vi "GPI-Movie merge.vi"() -> ()   [LabVIEW 2011]
doc: "Makes merged pseudo-color stills or movies from microscope images collected at two different wavelengths. Can handle either simultaneous or sequential multiwavelength acquisitions. The program uses the Matlab image registration tools to do the image alignments; these tools require the user to pick control points manually by mouse clicking. The images used to pick control points can be the images of the experiment or separate control images of a registration sample. The program handles tiffs or tiff stacks for stills; movies must be tiff stacks."
panel:
  in  "About":bool
  in  "Make a Movie":bool
  in  "Read Alignment Info from File":bool
  in  "Save Alignment Info to File":bool
  in  "View Alignment Images and Select Control Points":bool
  out "error out":errorcluster
  in  "Make a Merged Still Image and adjust intensities":bool
  in  "stop":bool
  in  "error in (no error)":errorcluster
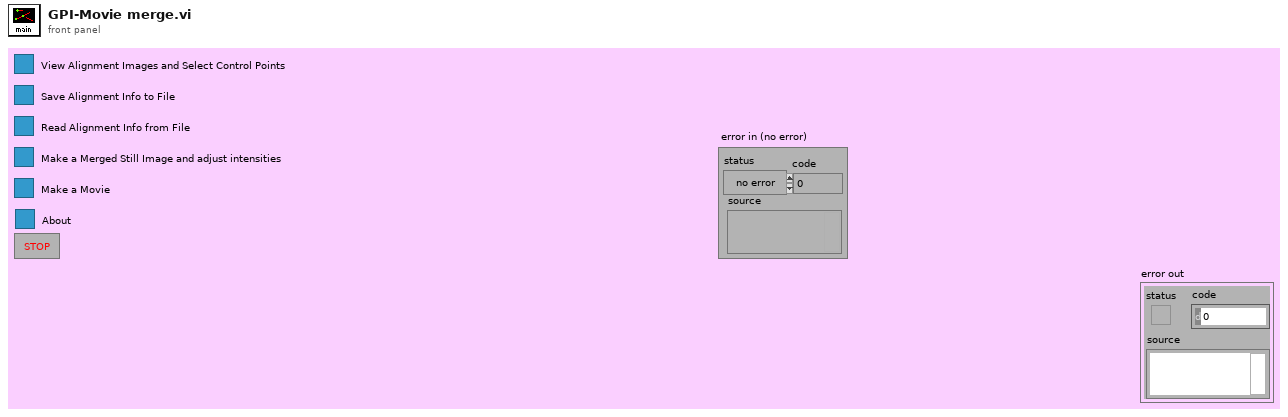
[diagram p1: front panel]
types:
  T1 = cluster{"File name":path, "TIFF stack?":bool, "Frame # if stack?":u32}[]
  T2 = typedef "IMAQ Image.ctl" = refnum<image>
  T3 = cluster{"Image Type":u32, "Image":T2, "Initialized?":bool, "Window Title":string, "Auto resize?":bool, "Auto position?":bool, "Autoscale?":bool, "Black/White Levels":cluster{ext, ext}, "Scale Min":ext, "Scale Max":ext}[]
  T4 = enum32{"existing file", "new file", "new or existing file", "existing dir", "new dir", "new or existing dir", "existing file (use LLBs)", "new file (use LLBs)", "new or existing file (use LLBs)", "new or existing file or directory (use LLBs)"}
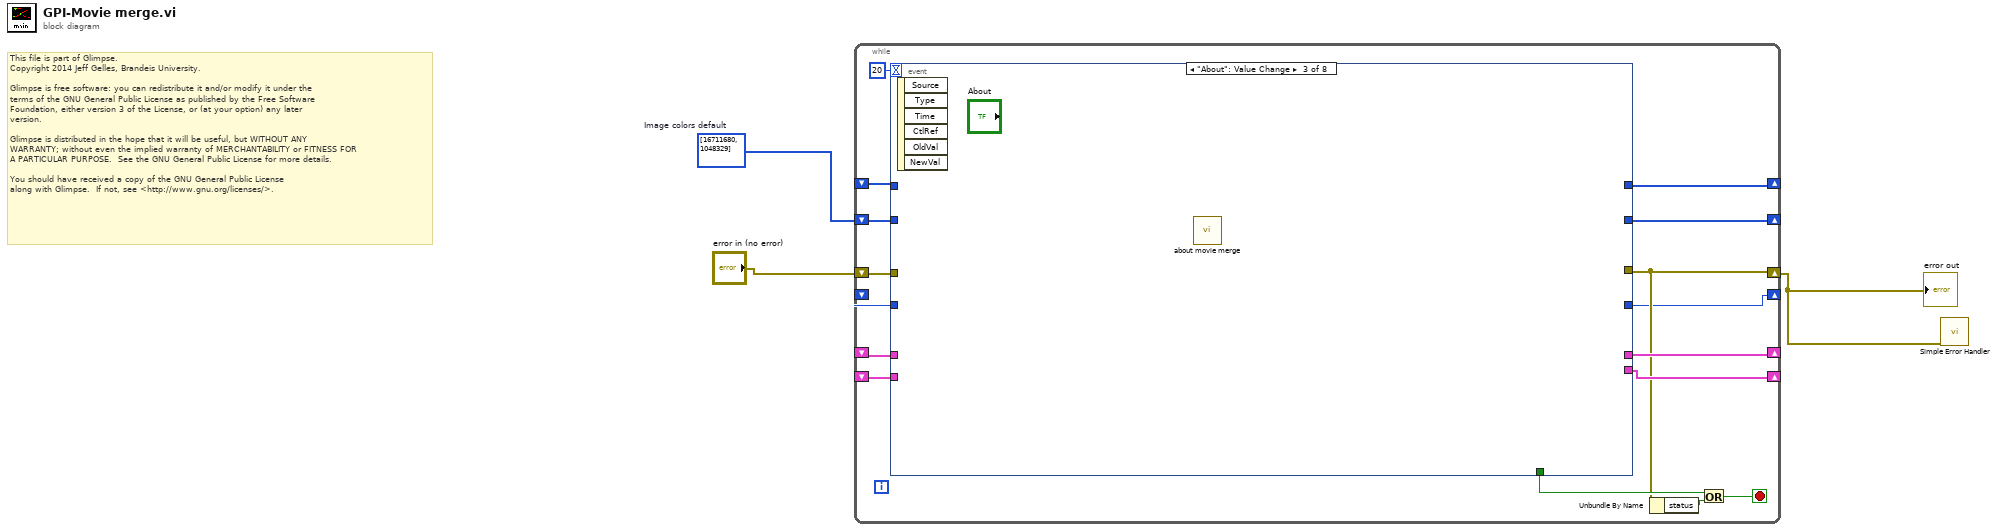
[diagram p0: block diagram]
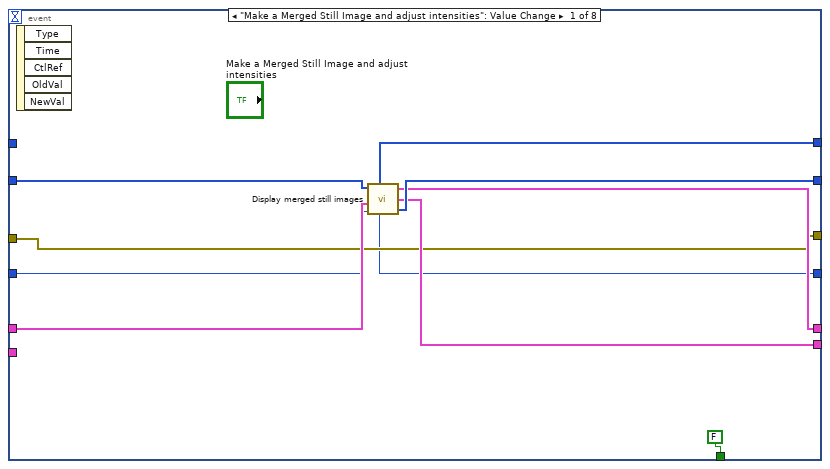
[diagram p2: hidden frame]
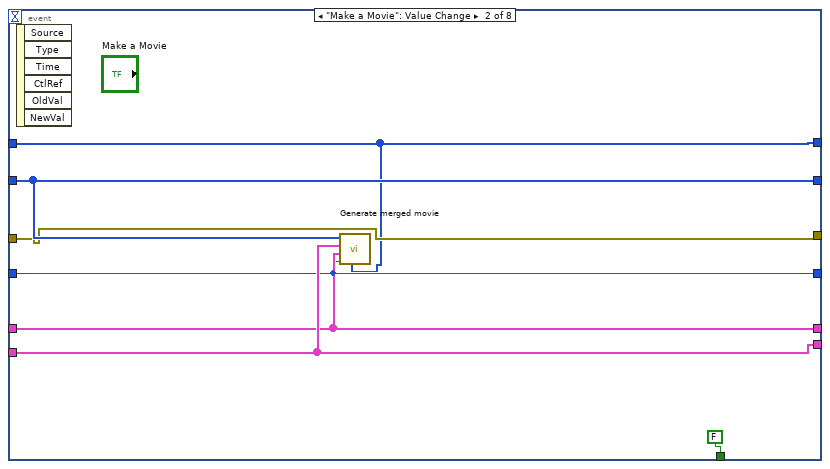
[diagram p3: hidden frame]
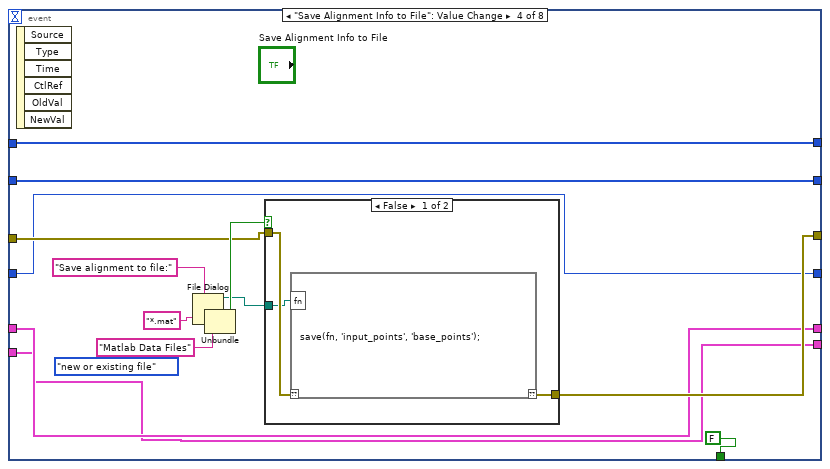
[diagram p4: hidden frame]
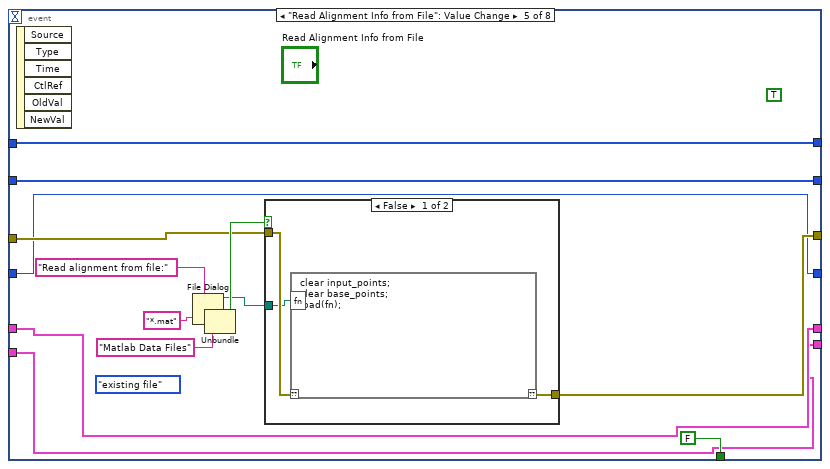
[diagram p6: hidden frame]
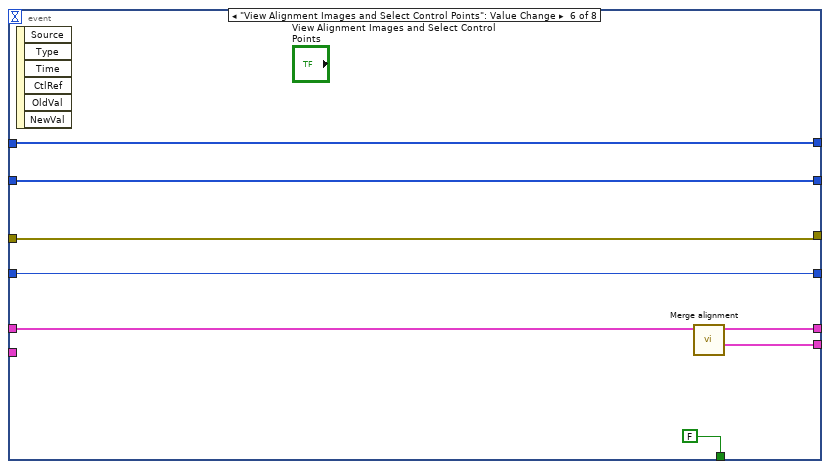
[diagram p8: hidden frame]
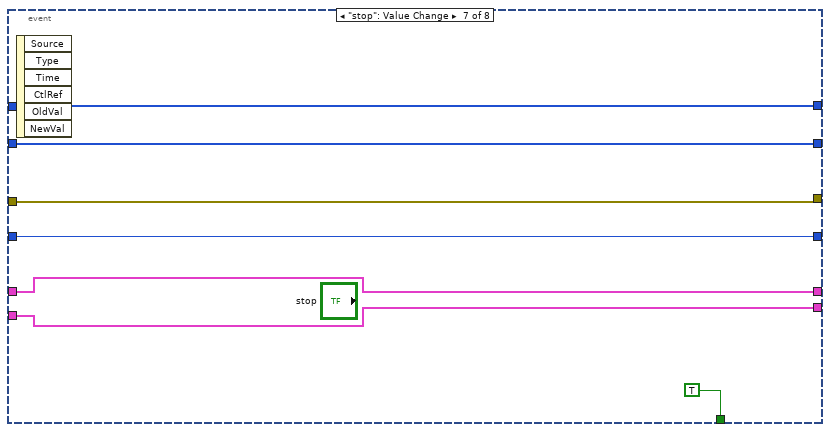
[diagram p9: hidden frame]
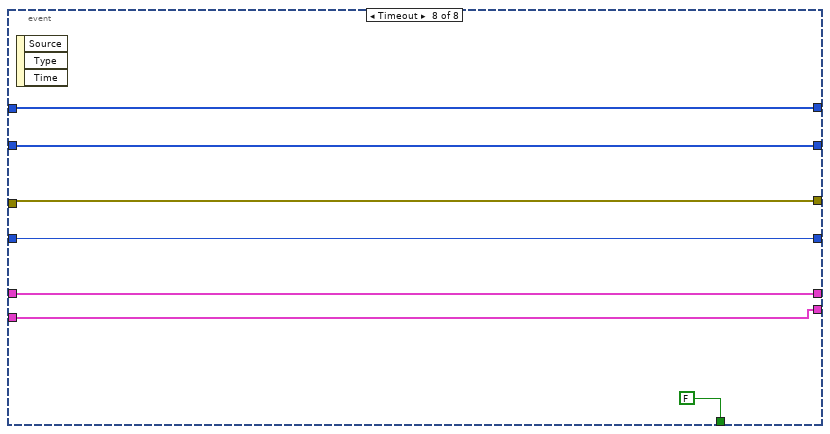
[diagram p10: hidden frame]
diagram:
  w1 = u32[] [16711680, 1048329]  # Image colors default
  # "This file is part of Glimpse. \nCopyright 2014 Jeff Gelles, Brandeis University.    \n\nGlimpse is free software: you can redistribute it and/or modify it under the \nterms of the GNU General Public License as published by the Free Software \nFoundation, either version 3 of the License, or (at your option) any later \nversion.\n\nGlimpse is distributed in the hope that it will be useful, but WITHOUT ANY \nWARRANTY; without even the implied warranty of MERCHANTABILITY or FITNESS FOR \nA PARTICULAR PURPOSE.  See the GNU General Public License for more details.\n\nYou should have received a copy of the GNU General Public License\nalong with Glimpse.  If not, see <http://www.gnu.org/licenses/>."
  n1 = while {
    shift-right: [w8] -> w2
    shift-left: "error in (no error)" -> [w15]
    shift-right: [w14] -> _
    shift-left: _ -> [w12]
    shift-right: [w13] -> _
    shift-left: _ -> [w11]
    shift-right: [w10] -> _
    shift-left: w1 -> [w9]
    shift-right: [w6] -> _
    shift-left: _ -> [w7]
    shift-right: [w5] -> _
    shift-left: _ -> [w4]
    stop <- w19 stop-if-true
    n2 = event shown="[2] \"About\": Value Change" {
      selector: _ -> [_ _ _ _ _ _ _ _]
      dyn-events: _ -> [_ _ _ _ _ _ _ _]
      timeout: 20 -> [_ _ _ _ _ _ _ _]
      tunnel: [FALSE ("stop") FALSE ("stop") _ FALSE ("stop") FALSE ("stop") FALSE ("stop") TRUE FALSE ("stop")] -> w18
      tunnel: w15 -> [w23 w33 _ w43 w61 w75 w86 w93]
      tunnel: [w23 w33 _ w45 w63 w75 w86 w93] -> w8
      tunnel: [w26 w35 _ w42 w60 w79 w85 w91] -> w14
      tunnel: [w25 w36 _ w41 w59 w78 w84 w90] -> w13
      tunnel: w12 -> [w24 w35 _ w42 w60 w77 w85 w91]
      tunnel: w11 -> [_ w36 _ w41 w59 _ w84 w90]
      tunnel: [w28 w34 _ w40 w58 w76 w83 w92] -> w10
      tunnel: w9 -> [w27 w34 _ w40 w58 w76 w83 w92]
      tunnel: w7 -> [w21 w32 _ w39 w57 w74 w82 w89]
      tunnel: [w22 w32 _ w39 w57 w74 w82 w89] -> w6
      tunnel: [w20 w31 _ w38 w56 w73 w81 w88] -> w5
      tunnel: w4 -> [_ w31 _ w38 w56 w73 w81 w88]
      event "Make a Merged Still Image and adjust intensities": Value Change {
        n3 = event-data() -> ()  [unwired: 6 out]
        n4 = call "Display merged still images.vi"("Image colors"=w27, "Image info"=w24, "Transform"=w21) -> ("ROI Out"=w20:i32[], "Transform out"=w22:u16, "Image info Out"=w26:T1, "Display info out"=w25:T3, "Image colors out"=w28:u32[])  [unwired: 1 out]
      }
      event "Make a Movie": Value Change {
        n5 = event-data() -> ()  [unwired: 7 out]
        n6 = call "Generate merged movie.vi"("Image colors"=w34, "Display info in"=w36, "Image info"=w35, "ROI"=w31, "Transform"=w32) -> ()  [unwired: 4 out]
      }
      event "About": Value Change {
        n7 = event-data() -> ()  [unwired: 7 out]
        n8 = call "about movie merge.vi"() -> ()  [unwired: 1 out]
      }
      event "Save Alignment Info to File": Value Change {
        (unwired) T4."new or existing file" ("select mode (2)")
        n9 = event-data() -> ()  [unwired: 7 out]
        n10 = File Dialog(4:"Matlab Data Files" ("pattern label"), 6:"*.mat" ("pattern"), 7:"Save alignment to file:" ("prompt")) -> (0:w37:errorcluster, 1:w47:bool, 3:w46:path)  [unwired: 1 in, 4 out]
        n11 = Unbundle(w37) -> ()  [unwired: 3 out]
        n12 = case shown="False" w47 {
          tunnel: w43 -> [w53 w54]
          tunnel: w46 -> [w52 _]
          tunnel: [w51 w54] -> w45
          frame False {
            n13 = script code="save(fn, 'input_points', 'base_points');"("??"=w53, "fn"=w52) -> ("??"=w51:errorcluster)
          }
          frame True {
          }
        }
      }
      event "Read Alignment Info from File": Value Change {
        (unwired) T4."existing file" ("select mode (2)")
        (unwired) TRUE
        n14 = event-data() -> ()  [unwired: 7 out]
        n15 = File Dialog(4:"Matlab Data Files" ("pattern label"), 6:"*.mat" ("pattern"), 7:"Read alignment from file:" ("prompt")) -> (0:w55:errorcluster, 1:w65:bool, 3:w64:path)  [unwired: 1 in, 4 out]
        n16 = Unbundle(w55) -> ()  [unwired: 3 out]
        n17 = case shown="False" w65 {
          tunnel: w61 -> [w71 w72]
          tunnel: w64 -> [w70 _]
          tunnel: [w69 w72] -> w63
          frame False {
            n18 = script code="clear input_points;\nclear base_points;\nload(fn);"("??"=w71, "fn"=w70) -> ("??"=w69:errorcluster)
          }
          frame True {
          }
        }
      }
      event "View Alignment Images and Select Control Points": Value Change {
        n19 = event-data() -> ()  [unwired: 7 out]
        n20 = call "Merge alignment.vi"("Image info"=w77) -> ("Display info out"=w78:T3, "Image info Out"=w79:T1)  [unwired: 6 out]
      }
      event "stop": Value Change {
        n21 = event-data() -> ()  [unwired: 7 out]
      }
      event Timeout {
        n22 = event-data() -> ()  [unwired: 4 out]
      }
    }
    n23 = Unbundle By Name(w8) -> ("status"=w17:bool)
    n24 = Or(x=w18, y=w17) -> (x .or. y?=w19:bool)
  }
  "error out" <- w2
  n25 = call <vilib>:"Simple Error Handler.vi"("error in (no error)"=w2) -> ()  [unwired: 1 in, 8 out]
